vi "TW Fix gRPC Register Dependencies.vi"(8 "error in":errorcluster, 9 "gRPC Service Name":string, 10 "Project Path":path, 11 "VI Refnum":refnum<vi>) -> (0 "error out":errorcluster)   [LabVIEW 2021, in "Plugin Generator.lvlib"]
uses:
  Plugin Generator.lvlib
  <vilib>/Utility/traverseref.llb/TRef TravTarget.ctl
  <vilib>/Utility/traverseref.llb/VI Scripting - Traverse.lvlib
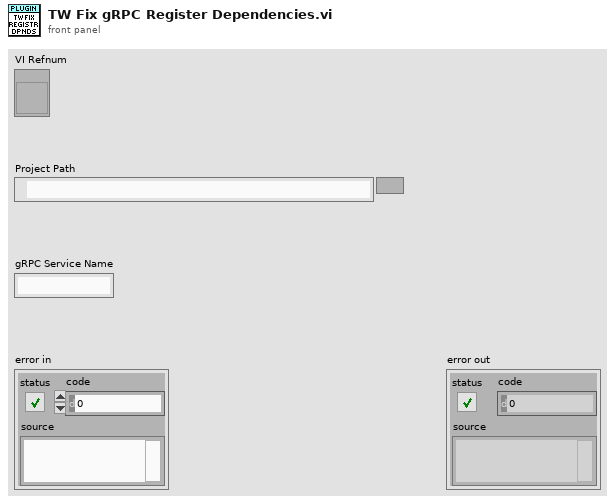
[diagram p1: front panel]
types:
  T1 = typedef "TRef TravTarget.ctl" = enum16{"FP", "BD", "Other"}
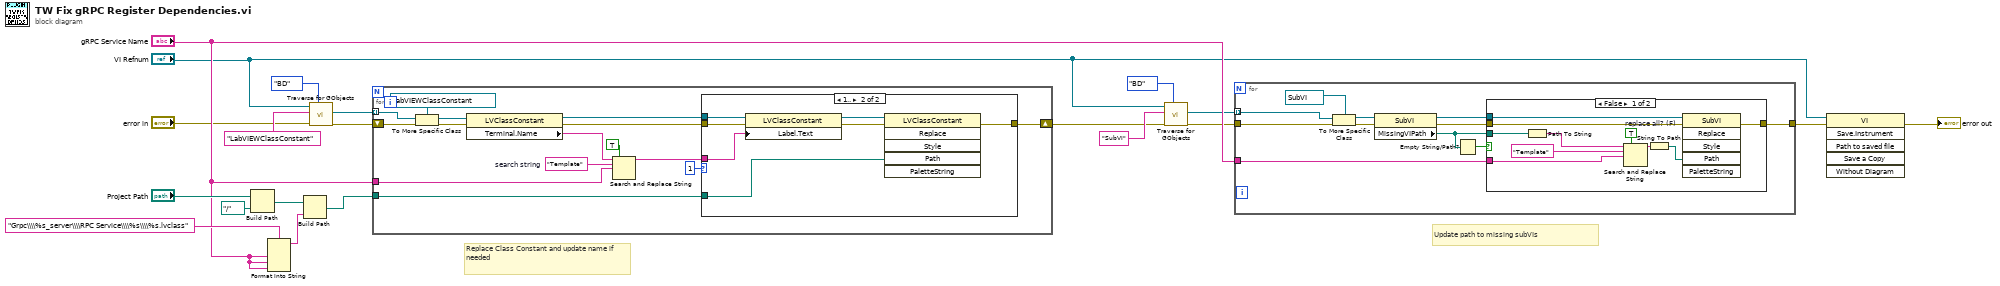
[diagram p0: block diagram]
diagram:
  # "Update path to missing subVIs"
  # "Replace Class Constant and update name if needed"
  n1 = Build Path(base path="Project Path", name or relative path=path "../..") -> (appended path=w13:path)
  n2 = Format Into String(format string="Grpc\\\\%s_server\\\\RPC Service\\\\%s\\\\%s.lvclass" ("Class Name"), "gRPC Service Name", "gRPC Service Name", "gRPC Service Name") -> (resulting string=w16:string)  [unwired: 2 in, 1 out]
  n3 = Build Path(base path=w13, name or relative path=w16) -> (appended path=w3:path)
  n4 = call <vilib>:"Traverse for GObjects.vi"("Traverse Target"=TRef_TravTarget."BD", "error in (no error)"="error in", "Class Name"="LabVIEWClassConstant", "VI Refnum"="VI Refnum") -> ("error out"=w10:errorcluster, "References"=w19:refnum<vi>[])  [unwired: 4 in, 2 out]
  n5 = for {
    tunnel: w19 -> [w35] mode=indexing
    tunnel: "gRPC Service Name" -> [w27]
    shift-right: [w30] -> w4
    shift-left: w10 -> [w23]
    tunnel: w3 -> [w22]
    w28 = "Template"  # search string
    n6 = To More Specific Class(target class=refnum<vi> refnum ("x"), reference=w35, error in=w23) -> (specific class reference=w29:refnum<vi>, error out=w33:errorcluster)
    n7 = property class="LVClassConstant"(reference=w29, error in=w33) -> (reference out=w31:refnum<vi>, error out=w32:errorcluster, "Terminal.Name"=w24:string)
    n8 = Search and Replace String(replace all?=TRUE ("replace all? (F)"), input string=w24, search string=w28, replace string=w27) -> (result string=w26:string)  [unwired: 4 in, 3 out]
    n9 = case shown="1.." 1 ("number of replacements") {
      tunnel: w32 -> [w36 w40]
      tunnel: w31 -> [_ w43]
      tunnel: [w36 w39] -> w30
      tunnel: w26 -> [_ w38]
      tunnel: w22 -> [_ w37]
      frame 0, Default {
      }
      frame 1.. {
        n10 = property class="LVClassConstant"(reference=w43, error in=w40, "Label.Text"=w38) -> (reference out=w42:refnum<vi>, error out=w41:errorcluster)
        n11 = invoke class="LVClassConstant" method="Replace"(reference=w42, error in=w41, "Path"=w37) -> (error out=w39:errorcluster)  [unwired: 3 in, 5 out]
      }
    }
  }
  n12 = call <vilib>:"Traverse for GObjects.vi"("Traverse Target"=TRef_TravTarget."BD", "error in (no error)"=w4, "Class Name"="SubVI", "VI Refnum"="VI Refnum") -> ("error out"=w5:errorcluster, "References"=w6:refnum<vi>[])  [unwired: 4 in, 2 out]
  n13 = for {
    tunnel: w6 -> [w46] mode=indexing
    tunnel: "gRPC Service Name" -> [w51]
    tunnel: w5 -> [w49]
    tunnel: [w44] -> w11
    n14 = To More Specific Class(target class=refnum<vi> refnum ("x"), reference=w46, error in=w49) -> (specific class reference=w47:refnum<vi>, error out=w45:errorcluster)
    n15 = property class="SubVI"(reference=w47, error in=w45) -> (reference out=w53:refnum<vi>, error out=w50:errorcluster, "MissingVIPath"=w52:path)
    n16 = Empty String/Path?(string/path=w52) -> (empty?=w54:bool)
    n17 = case shown="False" w54 {
      tunnel: w53 -> [w64 _]
      tunnel: w52 -> [w62 _]
      tunnel: w51 -> [w58 _]
      tunnel: w50 -> [w56 w65]
      tunnel: [w55 w65] -> w44
      frame False {
        w57 = TRUE  # replace all? (F)
        n18 = Path To String(path=w62) -> (string=w63:string)
        n19 = Search and Replace String(replace all?=w57, input string=w63, search string="Template", replace string=w58) -> (result string=w60:string)  [unwired: 4 in, 3 out]
        n20 = String To Path(string=w60) -> (path=w59:path)
        n21 = invoke class="SubVI" method="Replace"(reference=w64, error in=w56, "Path"=w59) -> (error out=w55:errorcluster)  [unwired: 3 in, 5 out]
      }
      frame True {
      }
    }
  }
  n22 = invoke class="VI" method="Save.Instrument"(reference="VI Refnum", error in=w11) -> (error out=→"error out":errorcluster)  [unwired: 4 in, 5 out]
